vi "get_string_value.vi"(3 "error in (no error)":errorcluster, 4 "field name":string, 5 "metadata JSON string":string) -> (0 "error out":errorcluster, 2 "field value":string)   [LabVIEW 2013]
uses:
  <vilib>/LVH/i3 JSON/JSON Parsing/Get Object Parameter Files/Get Object Parameter - String.vi
  i3 JSON/i3-json.lvlib
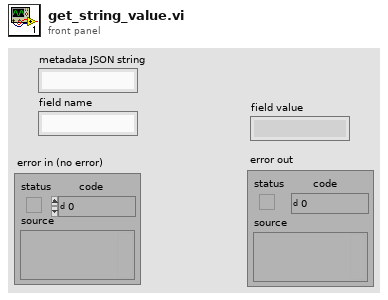
[diagram p1: front panel]
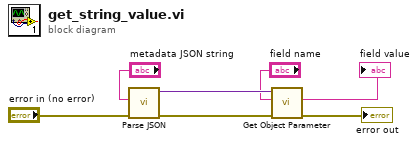
[diagram p0: block diagram]
diagram:
  n1 = call <vilib>:"Parse JSON.vi"("error in (no error)"="error in (no error)", "JSON String"="metadata JSON string") -> ("error out"=w2:errorcluster, "JSON Tree"=w7:variant)  [unwired: 6 in, 2 out]
  n2 = call-poly <vilib>:"Get Object Parameter.vi"("error in (no error)"=w2, "Parameter Name"="field name", "JSON Tree In (JSON Object)"=w7) -> ("error out"=→"error out":errorcluster, "String Value"=→"field value":string)  [unwired: 5 in, 2 out]
